vi "Sample_String_Splitter.vi"(7 "Sample String":string) -> (2 "Sample Number":string, 3 "Sample Name":string)   [LabVIEW 2022 SP3]
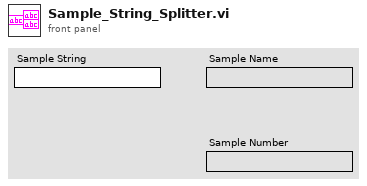
[diagram p1: front panel]
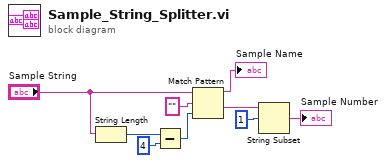
[diagram p0: block diagram]
diagram:
  n1 = String Length(string="Sample String") -> (length=w2:i32)
  n2 = Subtract(x=w2, y=4) -> (x-y=w4:i32)
  n3 = Match Pattern(string="Sample String", regular expression="", offset (0)=w4) -> (before substring=→"Sample Name":string, after substring=w7:string)  [unwired: 2 out]
  n4 = String Subset(string=w7, offset (0)=1) -> (substring=→"Sample Number":string)  [unwired: 1 in]
